vi "Get Classes in Memory.vi"(8 "error in (no error)":errorcluster, 11 "Class Name in (*.lvclass)":string) -> (0 "error out":errorcluster, 1 "Found?":bool, 2 "Children (*.lvclass)":string[](array[string]), 3 "Parents (*.lvclass)":string[](array[string]), 5 "All Classes in Memory":T1(array[cluster]))   [LabVIEW 2018]
doc: "Returns the parent and child classes in memory given qualified Class Name in (*.lvclass)."
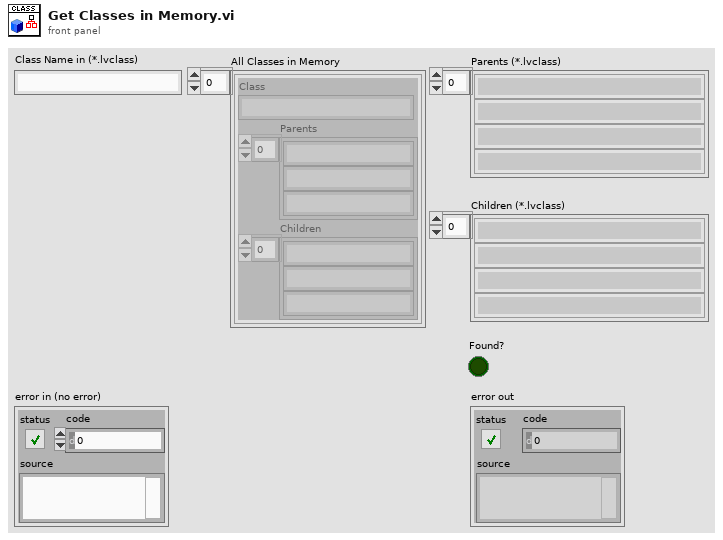
[diagram p1: front panel]
types:
  T1 = cluster{"Class":string, "Parents":string[], "Children":string[]}[]
  T2 = cluster{"Self":i32, "Parents":i32[], "Children":i32[]}
  T3 = cluster{"Self":i32, "Parents":i32[], "Children":i32[]}[]
  T4 = cluster{"Class":string, "Parents":string[], "Children":string[]}
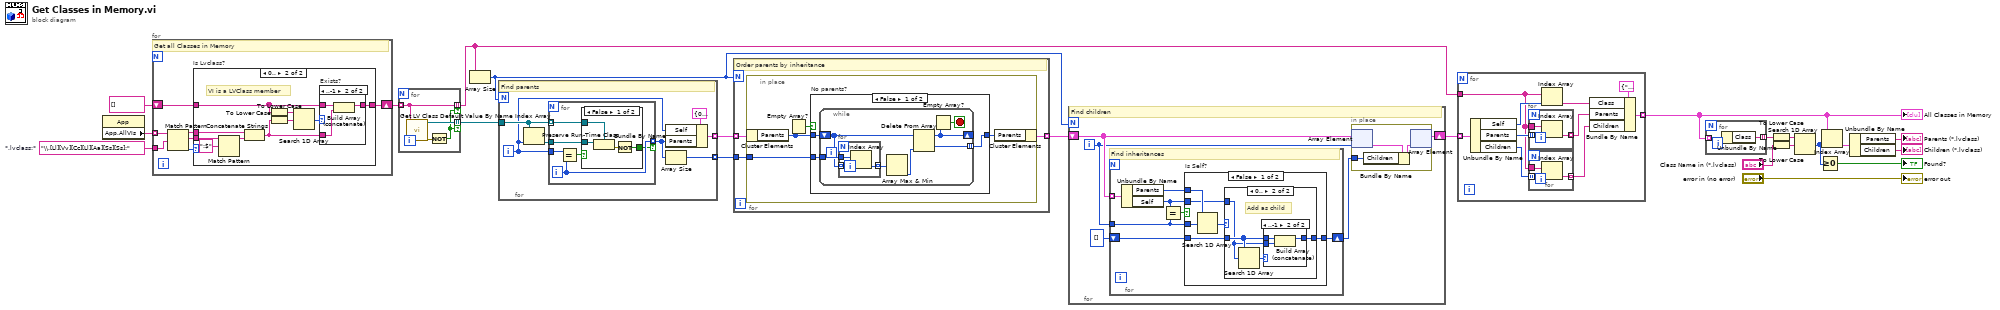
[diagram p0: block diagram]
diagram:
  w13 = "\\.[Ll][Vv][Cc][Ll][Aa][Ss][Ss]:"  # *.lvclass:*
  n1 = property class="App"() -> ("App.AllVIs"=w12:string[])  [unwired: 2 in, 2 out]
  n2 = for {
    tunnel: w12 -> [w29] mode=indexing
    tunnel: w13 -> [w28]
    shift-right: [w24] -> w16
    shift-left: string[] [] ("Application:All VIs In Memory") -> [w25]
    # "Get all Classes in Memory"
    n3 = Match Pattern(string=w29, regular expression=w28) -> (before substring=w27:string, match substring=w26:string, offset past match=w23:i32)  [unwired: 1 in, 1 out]
    n4 = case "Is Lvclass?" shown="0.." w23 {
      tunnel: w27 -> [_ w40]
      tunnel: w26 -> [_ w39]
      tunnel: w25 -> [w30 w34]
      tunnel: [w30 w32] -> w24
      frame ..-1 {
      }
      frame 0.. {
        # "VI is a LVClass member"
        n5 = Match Pattern(string=w39, regular expression=":$") -> (before substring=w38:string)  [unwired: 1 in, 3 out]
        n6 = Concatenate Strings(w40, w38) -> (w33:string)
        n7 = To Lower Case(string=w34) -> (all lower case string=w35:string[])
        n8 = To Lower Case(string=w33) -> (all lower case string=w36:string)
        n9 = Search 1D Array(1D array=w35, element=w36) -> (index of element=w31:i32)  [unwired: 1 in]
        n10 = case "Exists?" shown="..-1" w31 {
          tunnel: w34 -> [w41 w44]
          tunnel: w33 -> [_ w43]
          tunnel: [w41 w42] -> w32
          frame 0.. {
          }
          frame ..-1 {
            n11 = Build Array (concatenate)(w44, w43) -> (w42:string[])
          }
        }
      }
    }
  }
  n12 = for {
    tunnel: w16 -> [w46] mode=indexing
    tunnel: [w47] -> w22 mode=indexing if=w45
    tunnel: [w46] -> w15 mode=indexing if=w45
    n13 = call <vilib>:"Get LV Class Default Value By Name.vi"("class name"=w46) -> ("error out"=w48:errorcluster, "object"=w47:refnum<class>)  [unwired: 9 in]
    n14 = Not(x=w48) -> (.not. x?=w45:bool)
  }
  n15 = Array Size(array=w15) -> (size(s)=w18:i32)
  n16 = for {
    N: w18 -> [_]
    tunnel: w22 -> [w55]
    tunnel: [w52] -> w21 mode=indexing
    tunnel: [w50] -> w20 mode=indexing
    i -> [w49]
    # "Find parents"
    n17 = Index Array(array=w55, index=w49) -> (element=w54:refnum<class>)
    n18 = for {
      tunnel: w55 -> [w61] mode=indexing
      tunnel: w54 -> [w60]
      tunnel: w49 -> [w59]
      tunnel: [w57] -> w51 mode=indexing if=w56
      i -> [w57]
      n19 = Equal?(x=w59, y=w57) -> (x = y?=w58:bool)
      n20 = case shown="False" w58 {
        tunnel: w61 -> [w65 _]
        tunnel: w60 -> [w64 _]
        tunnel: [w62 _] -> w56
        frame False {
          n21 = Preserve Run-Time Class(object in=w64, 2:w65) -> (error out=w63:errorcluster)  [unwired: 1 in, 1 out]
          n22 = Not(x=w63) -> (.not. x?=w62:bool)
        }
        frame True {
        }
      }
    }
    n23 = Bundle By Name(cluster=T2 {"Self"=0, "Parents"=[], "Children"=[]} ("Inheritance"), "Self"=w49, "Parents"=w51) -> (w52:T2)
    n24 = Array Size(array=w51) -> (size(s)=w50:i32)
  }
  n25 = for {
    N: w18 -> [_]
    tunnel: w21 -> [w67] mode=indexing
    tunnel: w20 -> [w68]
    tunnel: [w66] -> w19 mode=indexing
    # "Order parents by inheritance"
    n26 = in-place {
      in-place-border: w68 -> [w71]
      n27 = in-place-cluster #1(w67) -> ("Parents"=w70:i32[])
      n28 = Empty Array?(array=w70) -> (empty?=w72:bool)
      n29 = case "No parents?" shown="False" w72 {
        tunnel: w70 -> [w75 w86]
        tunnel: w71 -> [w74 _]
        tunnel: [w73 w86] -> w69
        frame False {
          n30 = while {
            shift-right: [w78] -> _
            shift-left: w75 -> [w80]
            tunnel: w74 -> [w82]
            tunnel: [w76] -> w73 mode=indexing
            stop <- w77 stop-if-true
            n31 = for {
              tunnel: w82 -> [w85]
              tunnel: w80 -> [w84] mode=indexing
              tunnel: [w83] -> w81 mode=indexing
              n32 = Index Array(array=w85, index=w84) -> (element=w83:i32)
            }
            n33 = Array Max & Min(array=w81) -> (min index (indices)=w79:i32)  [unwired: 3 out]
            n34 = Delete From Array(array=w80, index=w79) -> (deleted portion=w76:i32, array with subset deleted=w78:i32[])  [unwired: 1 in]
            n35 = Empty Array?(array=w78) -> (empty?=w77:bool)
          }
        }
        frame True {
        }
      }
      n36 = in-place-cluster #1("Parents"=w69) -> (w66:T2)
    }
  }
  n37 = for {
    N: w18 -> [_]
    shift-right: [w88] -> w17
    shift-left: w19 -> [w90]
    i -> [w89]
    # "Find children"
    n38 = for {
      tunnel: w90 -> [w98] mode=indexing
      tunnel: w89 -> [w96]
      shift-right: [w93] -> w87
      shift-left: i32[] [] ("Children") -> [w94]
      # "Find inheritances"
      n39 = Unbundle By Name(w98) -> ("Parents"=w97:i32[], "Self"=w92:i32)
      n40 = Equal?(x=w92, y=w96) -> (x = y?=w95:bool)
      n41 = case "Is Self?" shown="False" w95 {
        tunnel: w97 -> [w103 _]
        tunnel: w96 -> [w104 _]
        tunnel: w94 -> [w102 w114]
        tunnel: [w101 w114] -> w93
        tunnel: w92 -> [w99 _]
        frame False {
          n42 = Search 1D Array(1D array=w103, element=w104) -> (index of element=w100:i32)  [unwired: 1 in]
          n43 = case shown="0.." w100 {
            tunnel: w102 -> [w105 w109]
            tunnel: [w105 w108] -> w101
            tunnel: w99 -> [_ w106]
            frame ..-1 {
            }
            frame 0.. {
              # "Add as child"
              n44 = Search 1D Array(1D array=w109, element=w106) -> (index of element=w107:i32)  [unwired: 1 in]
              n45 = case shown="..-1" w107 {
                tunnel: w109 -> [w110 w113]
                tunnel: [w110 w112] -> w108
                tunnel: w106 -> [_ w111]
                frame 0.. {
                }
                frame ..-1 {
                  n46 = Build Array (concatenate)(w113, w111) -> (w112:i32[])
                }
              }
            }
          }
        }
        frame True {
        }
      }
    }
    n47 = in-place {
      in-place-border: w87 -> [w115]
      n48 = in-place-array #2(w90, w89) -> (w117:T2)
      n49 = Bundle By Name(cluster=w117, "Children"=w115) -> (w116:T2)
      n50 = in-place-array #2(w116) -> (w88:T3)  [unwired: 1 out]
    }
  }
  n51 = for {
    tunnel: w17 -> [w127] mode=indexing
    tunnel: w15 -> [w122]
    tunnel: [w118] -> w7 mode=indexing
    n52 = Unbundle By Name(w127) -> ("Self"=w126:i32, "Parents"=w124:i32[], "Children"=w121:i32[])
    n53 = for {
      tunnel: w122 -> [w133]
      tunnel: w124 -> [w132] mode=indexing
      tunnel: [w131] -> w123 mode=indexing
      n54 = Index Array(array=w133, index=w132) -> (element=w131:string)
    }
    n55 = for {
      tunnel: w122 -> [w130]
      tunnel: w121 -> [w129] mode=indexing
      tunnel: [w128] -> w120 mode=indexing
      n56 = Index Array(array=w130, index=w129) -> (element=w128:string)
    }
    n57 = Index Array(array=w122, index=w126) -> (element=w125:string)
    n58 = Bundle By Name(cluster=T4 {"Class"="", "Parents"=[], "Children"=[]} ("Inheritance"), "Class"=w125, "Parents"=w123, "Children"=w120) -> (w118:T4)
  }
  "All Classes in Memory" <- w7
  n59 = for {
    tunnel: w7 -> [w135] mode=indexing
    tunnel: [w134] -> w11 mode=indexing
    n60 = Unbundle By Name(w135) -> ("Class"=w134:string)
  }
  n61 = To Lower Case(string=w11) -> (all lower case string=w8:string[])
  n62 = To Lower Case(string="Class Name in (*.lvclass)") -> (all lower case string=w9:string)
  n63 = Search 1D Array(1D array=w8, element=w9) -> (index of element=w4:i32)  [unwired: 1 in]
  n64 = Greater Or Equal To 0?(x=w4) -> (x >= 0?=→"Found?":bool)
  n65 = Index Array(array=w7, index=w4) -> (element=w6:T4)
  n66 = Unbundle By Name(w6) -> ("Parents"=→"Parents (*.lvclass)":string[], "Children"=→"Children (*.lvclass)":string[])
  "error out" <- "error in (no error)"
